vi "SubVI Function Call Parameters C Code Chunks.vi"(8 "Error In":errorcluster, 10 "VI Reference":refnum<vi>, 11 "SubVI Refnum":refnum<vi>) -> (0 "SubVI output variable name":string, 1 "SubVI func. declaration":string, 2 "return datatype":string, 3 "SubVI func. call in code":string, 4 "Error Out":errorcluster, 5 "reference out":refnum<vi>)   [LabVIEW 2014]
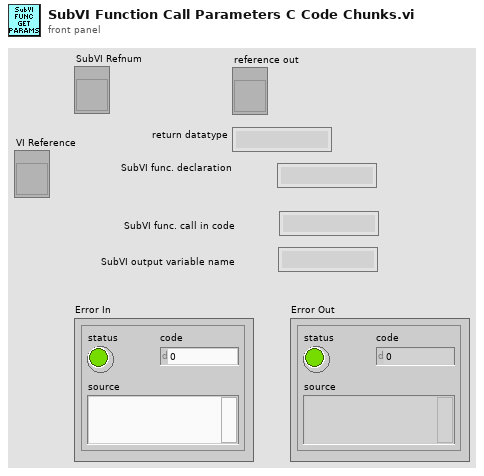
[diagram p1: front panel]
types:
  T1 = cluster{"terminals datatypes":string[][], "terminal\nconnected?":bool[], "terminal captions":string[], "term. count":i32, "terminal\nIsSource?":bool[], "SubVI name":string, "connected\nwires refs.":refnum<vi>[], "coerced dot?":bool[], "terminals[]":refnum<vi>[]}
  T2 = cluster{"wire labels":string[], "wire terminals datatypes":string[][]}
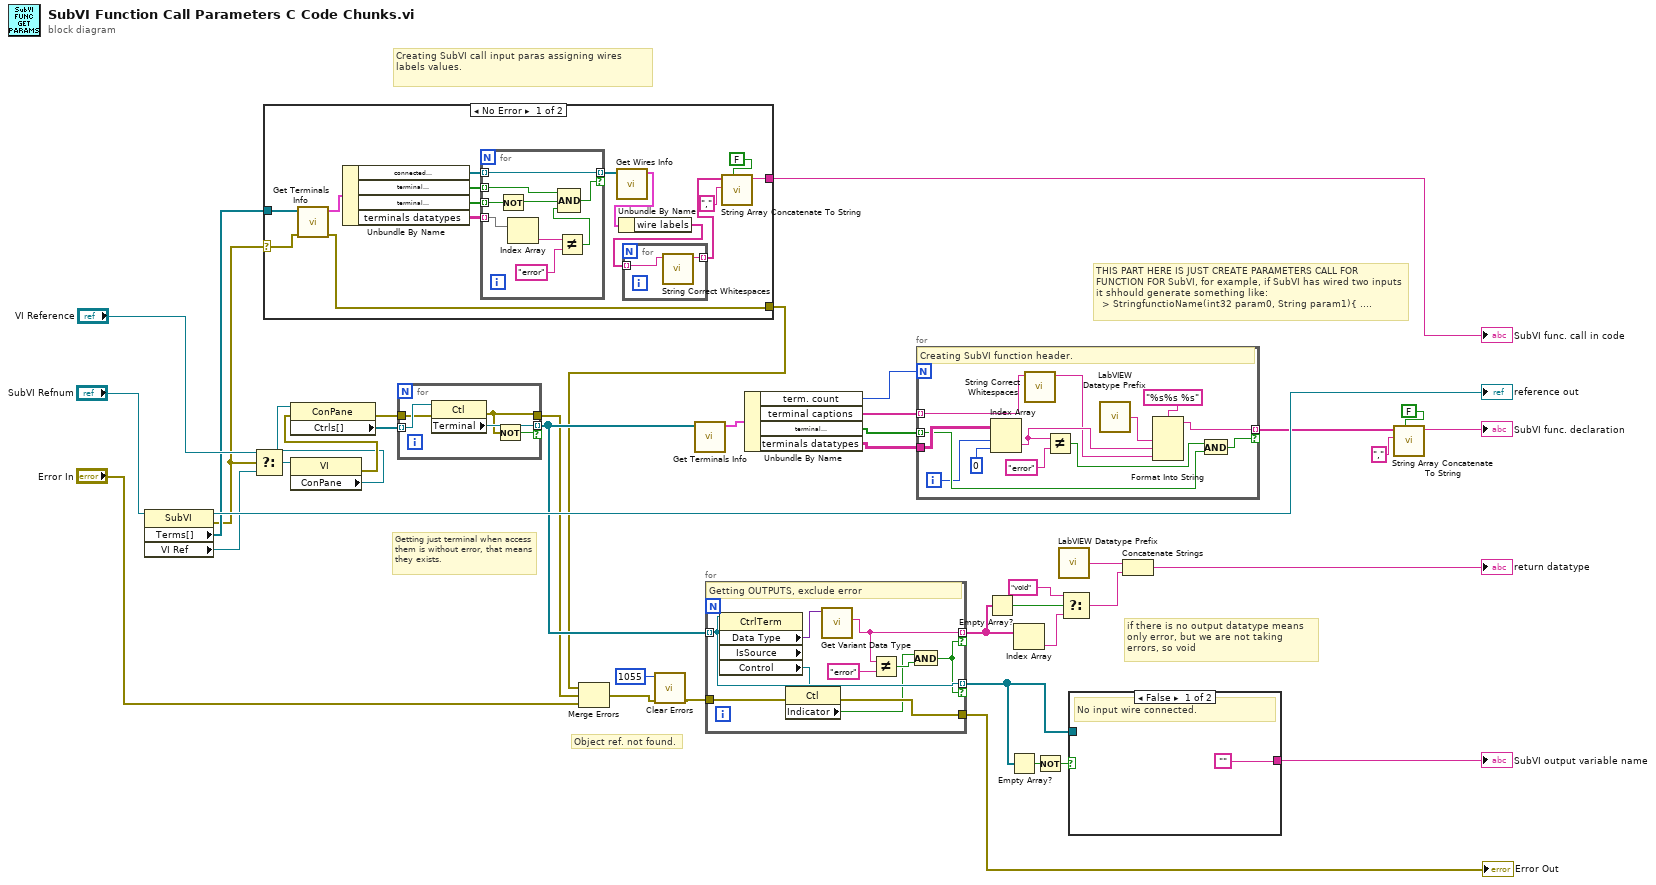
[diagram p0: block diagram]
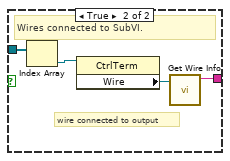
[diagram p3: hidden frame]
diagram:
  # "Getting just terminal when access them is without error, that means they exists."
  # "Object ref. not found."
  # "Creating SubVI call input paras assigning wires labels values."
  # "if there is no output datatype means only error, but we are not taking errors, so void"
  # "THIS PART HERE IS JUST CREATE PARAMETERS CALL FOR FUNCTION FOR SubVI, for example, if SubVI has wired two inputs it shhould generate something like:\n  > StringfunctioName(int32 param0, String param1){ ...."
  n1 = property class="SubVI"(reference="SubVI Refnum") -> (reference out=→"reference out":refnum<vi>, error out=w8:errorcluster, "Terms[]"=w9:refnum<vi>[], "VI Ref"=w11:refnum<vi>)  [unwired: 1 in]
  n2 = Select(t="VI Reference", s=w8, f=w11) -> (s? t:f=w10:refnum<vi>)
  n3 = case shown="No Error" w8 {
    selector: w8 -> [w42 w67]
    tunnel: w9 -> [w55 _]
    tunnel: [w43 _] -> w7
    tunnel: [w41 w67] -> w3
    frame No Error {
      n4 = call "Get Terminals Info.vi"("error in (no error)"=w42, "Terms[]"=w55) -> ("error out"=w41:errorcluster, "output cluster"=w54:T1)  [unwired: 8 in]
      n5 = Unbundle By Name(w54) -> ("connected\nwires refs."=w51:refnum<vi>[], "terminal\nconnected?"=w52:bool[], "terminal\nIsSource?"=w53:bool[], "terminals datatypes"=w50:string[][])
      n6 = for {
        tunnel: w53 -> [w66] mode=indexing
        tunnel: w52 -> [w64] mode=indexing
        tunnel: w51 -> [w63] mode=indexing
        tunnel: [w63] -> w48 mode=indexing if=w62
        tunnel: w50 -> [w60] mode=indexing
        n7 = Not(x=w66) -> (.not. x?=w65:bool)
        n8 = Index Array(array=w60) -> (element=w58:string)  [unwired: 1 in]
        n9 = Not Equal?(x=w58, y="error" ("x")) -> (x != y?=w61:bool)
        n10 = Compound Arithmetic op=AND(w64, w65, w61) -> (w62:bool)
      }
      n11 = call "Get Wires Info.vi"("connected\nwires refs."=w48) -> ("wires info cluster"=w49:T2)  [unwired: 10 in]
      n12 = Unbundle By Name(w49) -> ("wire labels"=w47:string[])
      n13 = for {
        tunnel: w47 -> [w57] mode=indexing
        tunnel: [w56] -> w44 mode=indexing
        n14 = call "String Correct Whitespaces.vi"("String in"=w57) -> ("String out"=w56:string)  [unwired: 10 in]
      }
      n15 = call "String Array Concatenate To String.vi"("insert last delimiter?"=FALSE, "Delimiter char"=",", "Array String In"=w44) -> ("String"=w43:string)  [unwired: 8 in]
    }
    frame Error {
    }
  }
  "SubVI func. call in code" <- w7
  n16 = property class="VI"(reference=w10) -> (error out=w16:errorcluster, "ConPane"=w15:refnum<vi>)  [unwired: 1 in, 1 out]
  n17 = property class="ConPane"(reference=w15, error in=w16) -> (error out=w6:errorcluster, "Ctrls[]"=w14:refnum<vi>[])  [unwired: 1 out]
  n18 = for {
    tunnel: w14 -> [w72] mode=indexing
    tunnel: [w71] -> w13 mode=indexing if=w70
    tunnel: w6 -> [w69]
    tunnel: [w68] -> w4
    n19 = property class="Ctl"(reference=w72, error in=w69) -> (error out=w68:errorcluster, "Terminal"=w71:refnum<vi>)  [unwired: 1 out]
    n20 = Not(x=w68) -> (.not. x?=w70:bool)
  }
  n21 = Merge Errors(w3, w4, "Error In") -> (w1:errorcluster)
  n22 = call <vilib>:"Clear Errors.vi"("error in (no error)"=w1, "specific error code to clear (0: all)"=1055) -> ("error out"=w2:errorcluster)  [unwired: 4 in, 1 out]
  n23 = call "Get Terminals Info.vi"("Terms[]"=w13) -> ("output cluster"=w22:T1)  [unwired: 9 in, 1 out]
  n24 = for {
    tunnel: [w80] -> w34 mode=indexing if=w76
    tunnel: w13 -> [w77] mode=indexing
    tunnel: [w77] -> w27 mode=indexing if=w76
    tunnel: [w75] -> w24
    tunnel: w2 -> [w75]
    # "Getting OUTPUTS, exclude error"
    n25 = property class="CtrlTerm" props=["Data Type", "IsSource", "Control"](reference=w77) -> ("Data Type"=w81:variant, "Control"=w74:refnum<vi>)  [unwired: 1 in, 3 out]
    n26 = property class="Ctl"(reference=w74) -> ("Indicator"=w73:bool)  [unwired: 1 in, 2 out]
    n27 = call "Get Variant Data Type.vi"("Variant in"=w81) -> ("first data type"=w80:string)  [unwired: 9 in, 1 out]
    n28 = Not Equal?(x=w80, y="error") -> (x != y?=w78:bool)
    n29 = And(x=w73, y=w78) -> (x .and. y?=w76:bool)
  }
  "Error Out" <- w24
  n30 = Unbundle By Name(w22) -> ("term. count"=w21:i32, "terminal captions"=w20:string[], "terminal\nIsSource?"=w19:bool[], "terminals datatypes"=w18:string[][])
  n31 = for {
    N: w21 -> [_]
    tunnel: w20 -> [w85] mode=indexing
    tunnel: w19 -> [w88] mode=indexing
    tunnel: w18 -> [w93]
    tunnel: [w90] -> w17 mode=indexing if=w83
    i -> [w82]
    # "Creating SubVI function header."
    n32 = Index Array(array=w93, index (row)=w82, index (col)=0 ("disabled index (col)")) -> (element=w87:string)
    n33 = call "String Correct Whitespaces.vi"("String in"=w85) -> ("String out"=w84:string)  [unwired: 10 in]
    n34 = Not Equal?(x=w87, y="error") -> (x != y?=w89:bool)
    n35 = call "LabVIEW Datatype Prefix.vi"() -> ("datatype prefix"=w86:string)
    n36 = Format Into String(format string="%s%s %s", w86, w87, w84) -> (resulting string=w90:string)  [unwired: 2 in, 1 out]
    n37 = And(x=w89, y=w88) -> (x .and. y?=w83:bool)
  }
  n38 = Empty Array?(array=w34) -> (empty?=w35:bool)
  n39 = Empty Array?(array=w27) -> (empty?=w28:bool)
  n40 = Index Array(array=w34) -> (element=w33:string)  [unwired: 1 in]
  n41 = Not(x=w28) -> (.not. x?=w26:bool)
  n42 = call "LabVIEW Datatype Prefix.vi"() -> ("datatype prefix"=w37:string)
  n43 = Select(t="void", s=w35, f=w33) -> (s? t:f=w31:string)
  n44 = case shown="False" w26 {
    tunnel: w27 -> [_ w99]
    tunnel: ["" w96] -> w29
    frame False {
      # "No input wire connected."
    }
    frame True {
      # "wire connected to output"
      # "Wires connected to SubVI."
      n45 = Index Array(array=w99) -> (element=w98:refnum<vi>)  [unwired: 1 in]
      n46 = property class="CtrlTerm"(reference=w98) -> ("Wire"=w97:refnum<vi>)  [unwired: 1 in, 2 out]
      n47 = call "Get Wire Info.vi"("Wire"=w97) -> ("wire label"=w96:string)  [unwired: 9 in, 1 out]
    }
  }
  "SubVI output variable name" <- w29
  n48 = Concatenate Strings(w37, w31) -> (→"return datatype":string)
  n49 = call "String Array Concatenate To String.vi"("insert last delimiter?"=FALSE, "Delimiter char"=",", "Array String In"=w17) -> ("String"=→"SubVI func. declaration":string)  [unwired: 8 in]
